vi "error_cluster.vi"() -> ()   [LabVIEW 2021]
panel:
  out "error out 2":errorcluster
  in  "error in (no error) 2":errorcluster
  out "error out":errorcluster
  in  "error in (no error)":errorcluster
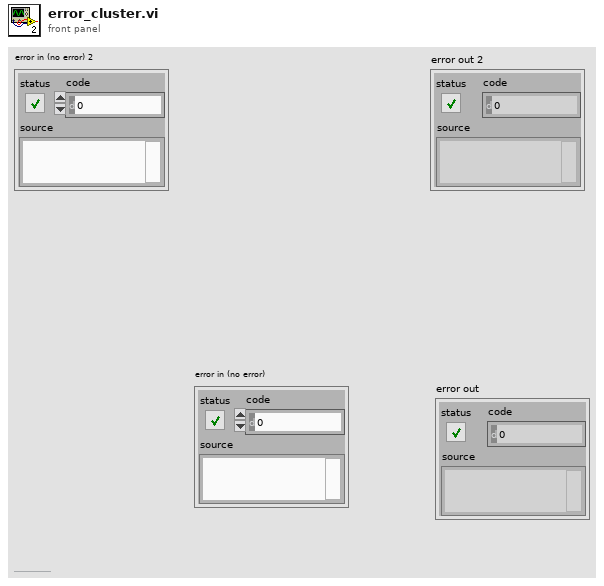
[diagram p1: front panel]
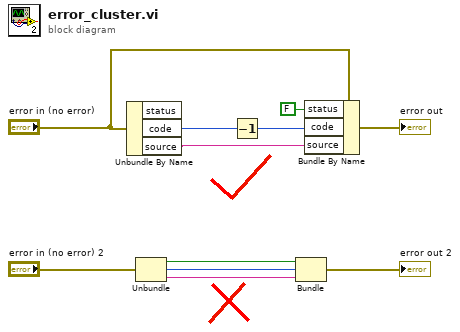
[diagram p0: block diagram]
diagram:
  n1 = Unbundle By Name "Unbundle By Name"("error in (no error)") -> ("code"=w9:i32, "source"=w6:string)  [unwired: 1 out]
  n2 = Unbundle "Unbundle"("error in (no error) 2") -> ("status"=w4:bool, "code"=w3:i32, "source"=w2:string)
  n3 = Decrement(x=w9) -> (x-1=w8:i32)
  n4 = Bundle "Bundle"("status"=w4, "code"=w3, "source"=w2) -> (→"error out 2":errorcluster)  [unwired: 1 in]
  n5 = Bundle By Name "Bundle By Name"(cluster="error in (no error)", "status"=FALSE, "code"=w8, "source"=w6) -> (→"error out":errorcluster)
